vi "AWG_5421_Run_And_Stop.vi"(8 "error  in":errorcluster caption="error in", 10 "Use Software trigger":bool, 11 "instrument handle in":refnum<k15>) -> (0 "error out":errorcluster)   [LabVIEW 2017]
doc: "I Description: FOR TESTS PURPOSE ONLY\nThis VI inits a waveform generation session for HSDIO 6541. This is a basic example that shows how to setup the board in order to generate waveforms according to a script. \n\nII Instructions for Running:\n1. Start the VI and select any previously created sequence script.\n2. If software trigger is choosen, just click on the Send Software Trigger button to generate the sequence.\nIf not, connect an external TTL trigger to the PFI0 input pin of the HSDIO, and generation will start immediately after the next trigger pulse.\n\nIII Block Diagram Steps:\n1. Initialize for a generation session.\n2. Assign the specified channels in Channel List for dynamic operation.\n3. Configure the Sample clock to use the onboard clock, and configure the clock rate.\n\n\n\n1. Initialize for a generation session.\n2. Assign specified channels in Channel List for dynamic operation : all = \"\" (default)\n3. Sets the Idle State for when the generation has completed : NO !!\n4. Configure the Sample clock to use the onboard clock, and configure the clock rate.\n5. Set generation mode to Scripted.\n6. Configure the Script Trigger : change to Digital Edge if waiting for an external\n trigger, and link Rising Edge and source trigger commands.\n Use PFI0 with SMB wired to the board, or any PFIxx if connected to accessory.\n6. Initiate dynamic pattern generation.\n7. Wait until the generation is done.\n8. Close the generation session."
uses:
  <instrlib>/niFgen/niFgen.llb/niFgen_ctl Trigger SW - TrigIdentifier Values (Ring).ctl
  <instrlib>/niFgen/niFgen.llb/niFgen_ctl Trigger SW - TrigName Values (Ring).ctl
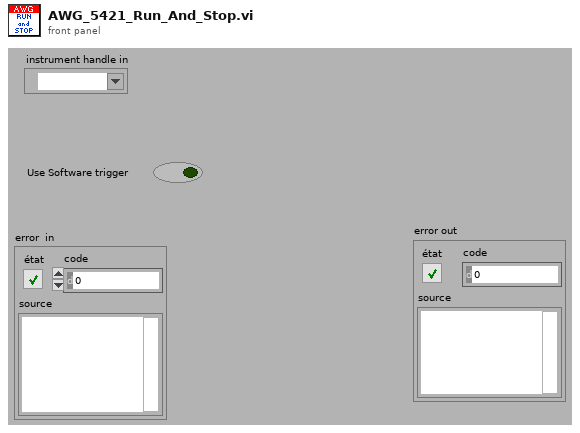
[diagram p1: front panel]
types:
  T1 = typedef "niFgen_ctl Trigger SW - TrigIdentifier Values (Ring).ctl" = string
  T2 = typedef "niFgen_ctl Trigger SW - TrigName Values (Ring).ctl" = i32
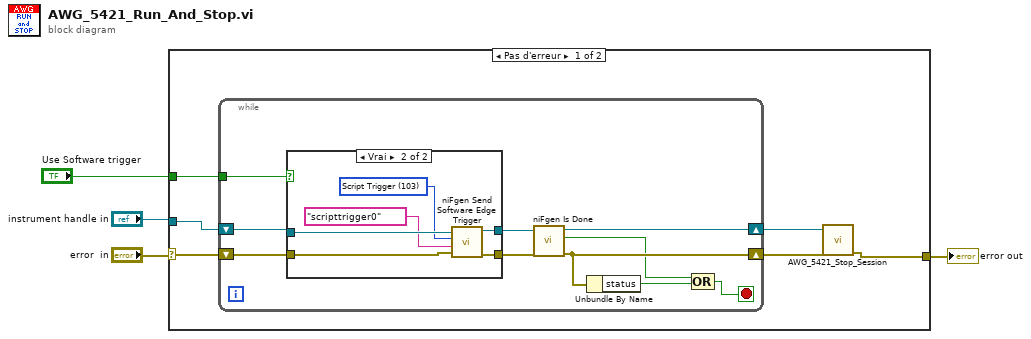
[diagram p0: block diagram]
diagram:
  n1 = case shown="Pas d'erreur" "error  in" {
    selector: "error  in" -> [w9 w29]
    tunnel: "instrument handle in" -> [w10 _]
    tunnel: [w5 w29] -> w4
    tunnel: "Use Software trigger" -> [w8 _]
    frame No Error {
      n2 = while {
        tunnel: w8 -> [w18]
        shift-right: [w15] -> w7
        shift-left: w10 -> [w20]
        shift-right: [w14] -> w6
        shift-left: w9 -> [w19]
        stop <- w11 stop-if-true
        n3 = case shown="Vrai" w18 {
          tunnel: [w21 w28] -> w17
          tunnel: [w22 w27] -> w16
          tunnel: w19 -> [w22 w26]
          tunnel: w20 -> [w21 w25]
          frame False {
          }
          frame True {
            w23 = T2 103 items=["Start Trigger"=1004, "Script Trigger"=103] ("Trigger (Start Trigger)")
            n4 = call <instrlib>:"niFgen Send Software Edge Trigger.vi"("error in (no error)"=w26, "Trigger ID (None)"=T1 "scripttrigger0", "Trigger (Start Trigger)"=w23, "Instrument Handle"=w25) -> ("error out"=w27:errorcluster, "Instrument Handle Out"=w28:refnum<k15>)  [unwired: 6 in]
          }
        }
        n5 = call <instrlib>:"niFgen Is Done.vi"("error in (no error)"=w16, "Instrument Handle"=w17) -> ("error out"=w14:errorcluster, "Done"=w13:bool, "Instrument Handle Out"=w15:refnum<k15>)  [unwired: 7 in]
        n6 = Unbundle By Name(w14) -> ("status"=w12:bool)
        n7 = Compound Arithmetic op=OR ("Opérateur arithmétique")(w13, w12) -> (w11:bool)
      }
      n8 = call "AWG_5421_Stop_Session.vi"("error in (no error)"=w6, "instrument handle in"=w7) -> ("error out"=w5:errorcluster)  [unwired: 9 in]
    }
    frame Error {
    }
  }
  "error out" <- w4
